vi "20150922_HW1_0412107_陳麒升.vi"() -> ()   [LabVIEW 2014]
panel:
  out "合成色-256RGB色碼總和":dbl(knob) scale=0.0..765.0
  out "合成色的R":dbl
  out "合成色的B":dbl
  out "合成色的G":dbl
  out "顏色2的R":dbl
  out "顏色2的B":dbl
  out "顏色2的G":dbl
  out "顏色1的R":dbl
  out "顏色1的B":dbl
  out "顏色1的G":dbl
  out "合成色(顏色1+顏色2)":u32(colorbox)
  out "合成色的B":i32 format="%x"
  out "合成色的G":i32 format="%x"
  out "合成色的R":i32 format="%x"
  out "顏色2-256RGB色碼總和":dbl(knob) scale=0.0..765.0
  in  "顏色2的B":i32 format="%x"
  in  "顏色2的G":i32 format="%x"
  in  "顏色2的R":i32 format="%x"
  out "顏色 2":u32(colorbox)
  out "顏色1-256RGB色碼總和":dbl(knob) scale=0.0..765.0
  out "顏色1":u32(colorbox)
  in  "顏色1的B":i32 format="%x"
  in  "顏色1的G":i32 format="%x"
  in  "顏色1的R":i32 format="%x"
  # "傳說中的網頁16進位色彩 ( hex color )調色盤"
  # "+"
  # "="
  # "16進位國際色碼"
  # "256RGB色碼"
  # "256RGB色碼"
  # "16進位國際色碼"
  # "256RGB色碼"
  # "16進位國際色碼"
  # "="
  # "+"
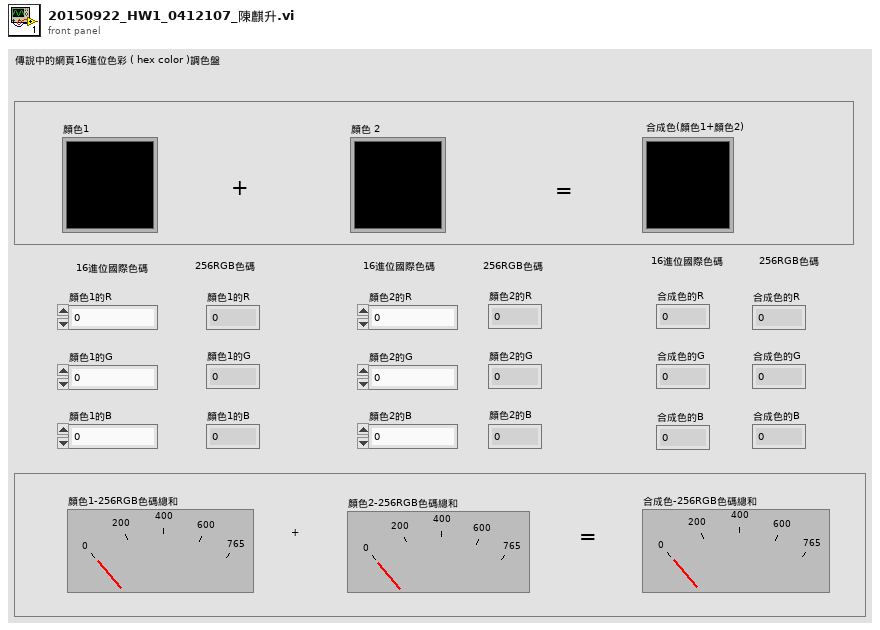
[diagram p1: front panel]
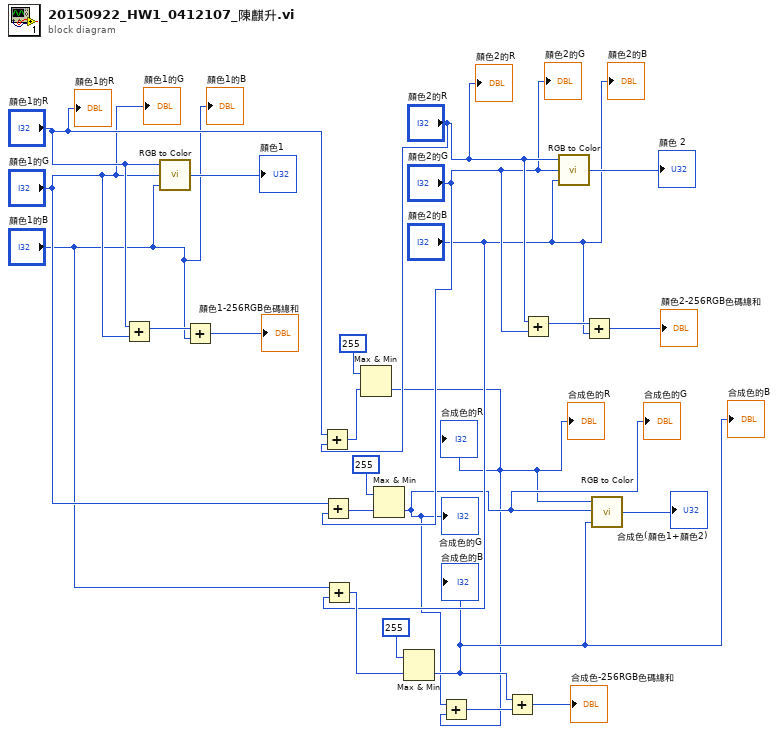
[diagram p0: block diagram]
diagram:
  n1 = Add(x="顏色1的R", y="顏色1的G") -> (x+y=w23:i32)
  n2 = call <vilib>:"RGB to Color.vi"("B"="顏色1的B", "G"="顏色1的G", "R"="顏色1的R") -> ("Color"=→"顏色1":u32)
  n3 = Add(x=w23, y="顏色1的B") -> (x+y=→"顏色1-256RGB色碼總和":i32)
  n4 = Add(x="顏色1的R", y="顏色2的R") -> (x+y=w16:i32)
  n5 = Add(x="顏色1的G", y="顏色2的G") -> (x+y=w14:i32)
  n6 = Add(x="顏色1的B", y="顏色2的B") -> (x+y=w12:i32)
  n7 = Max & Min(x=255, y=w16) -> (min(x,y)=w1:i32)  [unwired: 1 out]
  "合成色的R" <- w1
  "合成色的R" <- w1
  n8 = Max & Min(x=255, y=w14) -> (min(x,y)=w2:i32)  [unwired: 1 out]
  "合成色的G" <- w2
  "合成色的G" <- w2
  n9 = Max & Min(x=255, y=w12) -> (min(x,y)=w4:i32)  [unwired: 1 out]
  "合成色的B" <- w4
  "合成色的B" <- w4
  n10 = Add(x=w2, y=w1) -> (x+y=w3:i32)
  n11 = Add(x=w4, y=w3) -> (x+y=→"合成色-256RGB色碼總和":i32)
  n12 = Add(x="顏色2的R", y="顏色2的G") -> (x+y=w20:i32)
  n13 = call <vilib>:"RGB to Color.vi"("B"="顏色2的B", "G"="顏色2的G", "R"="顏色2的R") -> ("Color"=→"顏色 2":u32)
  n14 = Add(x=w20, y="顏色2的B") -> (x+y=→"顏色2-256RGB色碼總和":i32)
  n15 = call <vilib>:"RGB to Color.vi"("B"=w4, "G"=w2, "R"=w1) -> ("Color"=→"合成色(顏色1+顏色2)":u32)
  "顏色1的G" <- "顏色1的G"
  "顏色1的B" <- "顏色1的B"
  "顏色1的R" <- "顏色1的R"
  "顏色2的G" <- "顏色2的G"
  "顏色2的B" <- "顏色2的B"
  "顏色2的R" <- "顏色2的R"
